vi "Sensor handling scada.vi"(7 "connect (T)":bool=TRUE, 9 "color schema":i32 step=1, 10 "AI_ALRState":i32 step=1, 11 "AI_State":i32 step=1) -> (2 "ALRSTATE":errorcluster, 3 "STATE":T1)   [LabVIEW 2019, in "Inputs.lvlib"]
uses:
  Inputs.lvlib
  Ctl/Parameter State.ctl
  Ctl/Sensor alarm scada.ctl
  Ctl/Sensor state scada.ctl
  Alarms/Alarms.lvlib
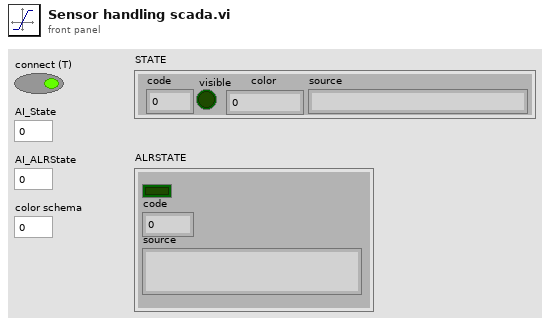
[diagram p1: front panel]
types:
  T1 = typedef "Inputs.lvlib/Parameter State.ctl" = cluster{"code":i32, "visible":bool, "color":u32, "source":string}
  T2 = typedef "Alarms.lvlib/Sensor alarm scada.ctl" = cluster{"source":string, "color":u32, "visible":bool}[]
  T3 = typedef "Inputs.lvlib/Sensor state scada.ctl" = cluster{"source":string, "color":u32, "visible":bool}[]
  T4 = cluster{"source":string, "color":u32, "visible":bool}
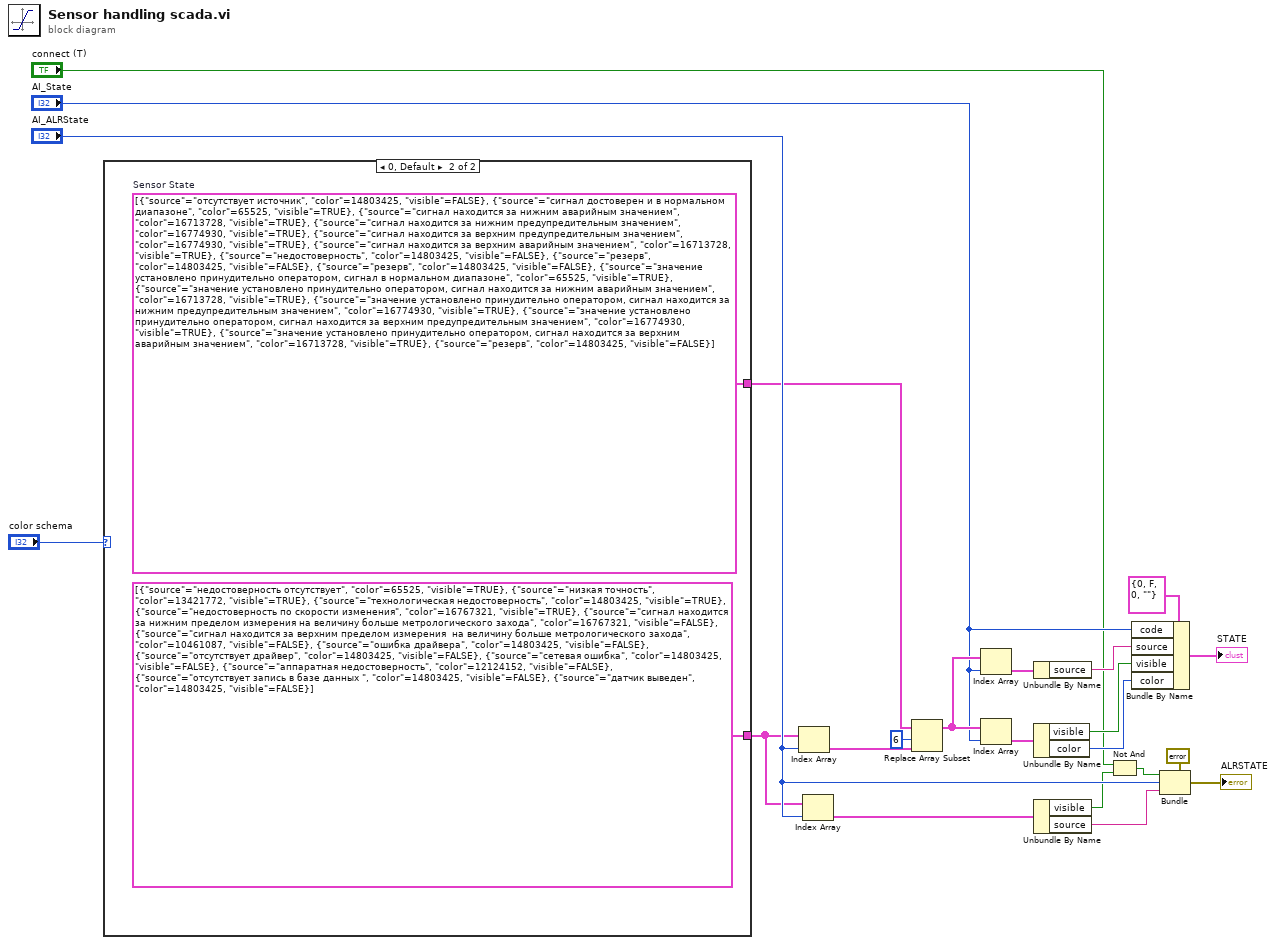
[diagram p0: block diagram]
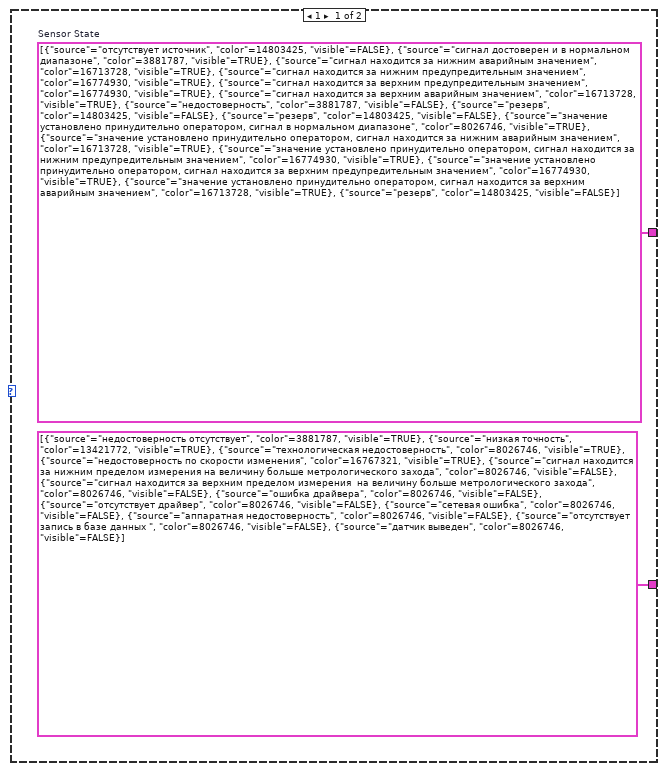
[diagram p2: hidden frame]
diagram:
  n1 = case shown="0, Default" "color schema" {
    tunnel: [w24 w26] -> w3
    tunnel: [T2 [{"source"="недостоверность отсутствует", "color"=3881787, "visible"=TRUE}, {"source"="низкая точность", "color"=13421772, "visible"=TRUE}, {"source"="технологическая недостоверность", "color"=8026746, "visible"=TRUE}, {"source"="недостоверность по скорости изменения", "color"=16767321, "visible"=TRUE}, {"source"="сигнал находится за нижним пределом измерения на величину больше метрологического захода", "color"=8026746, "visible"=FALSE}, {"source"="сигнал находится за верхним пределом измерения  на величину больше метрологического захода", "color"=8026746, "visible"=FALSE}, {"source"="ошибка драйвера", "color"=8026746, "visible"=FALSE}, {"source"="отсутствует драйвер", "color"=8026746, "visible"=FALSE}, {"source"="сетевая ошибка", "color"=8026746, "visible"=FALSE}, {"source"="аппаратная недостоверность", "color"=8026746, "visible"=FALSE}, {"source"="отсутствует запись в базе данных ", "color"=8026746, "visible"=FALSE}, {"source"="датчик выведен", "color"=8026746, "visible"=FALSE}] ("Array") T2 [{"source"="недостоверность отсутствует", "color"=65525, "visible"=TRUE}, {"source"="низкая точность", "color"=13421772, "visible"=TRUE}, {"source"="технологическая недостоверность", "color"=14803425, "visible"=TRUE}, {"source"="недостоверность по скорости изменения", "color"=16767321, "visible"=TRUE}, {"source"="сигнал находится за нижним пределом измерения на величину больше метрологического захода", "color"=16767321, "visible"=FALSE}, {"source"="сигнал находится за верхним пределом измерения  на величину больше метрологического захода", "color"=10461087, "visible"=FALSE}, {"source"="ошибка драйвера", "color"=14803425, "visible"=FALSE}, {"source"="отсутствует драйвер", "color"=14803425, "visible"=FALSE}, {"source"="сетевая ошибка", "color"=14803425, "visible"=FALSE}, {"source"="аппаратная недостоверность", "color"=12124152, "visible"=FALSE}, {"source"="отсутствует запись в базе данных ", "color"=14803425, "visible"=FALSE}, {"source"="датчик выведен", "color"=14803425, "visible"=FALSE}] ("Array")] -> w2
    frame 1 {
      w24 = T3 [{"source"="отсутствует источник", "color"=14803425, "visible"=FALSE}, {"source"="сигнал достоверен и в нормальном диапазоне", "color"=3881787, "visible"=TRUE}, {"source"="сигнал находится за нижним аварийным значением", "color"=16713728, "visible"=TRUE}, {"source"="сигнал находится за нижним предупредительным значением", "color"=16774930, "visible"=TRUE}, {"source"="сигнал находится за верхним предупредительным значением", "color"=16774930, "visible"=TRUE}, {"source"="сигнал находится за верхним аварийным значением", "color"=16713728, "visible"=TRUE}, {"source"="недостоверность", "color"=3881787, "visible"=FALSE}, {"source"="резерв", "color"=14803425, "visible"=FALSE}, {"source"="резерв", "color"=14803425, "visible"=FALSE}, {"source"="значение установлено принудительно оператором, сигнал в нормальном диапазоне", "color"=8026746, "visible"=TRUE}, {"source"="значение установлено принудительно оператором, сигнал находится за нижним аварийным значением", "color"=16713728, "visible"=TRUE}, {"source"="значение установлено принудительно оператором, сигнал находится за нижним предупредительным значением", "color"=16774930, "visible"=TRUE}, {"source"="значение установлено принудительно оператором, сигнал находится за верхним предупредительным значением", "color"=16774930, "visible"=TRUE}, {"source"="значение установлено принудительно оператором, сигнал находится за верхним аварийным значением", "color"=16713728, "visible"=TRUE}, {"source"="резерв", "color"=14803425, "visible"=FALSE}]  # Sensor State
    }
    frame 0, Default {
      w26 = T3 [{"source"="отсутствует источник", "color"=14803425, "visible"=FALSE}, {"source"="сигнал достоверен и в нормальном диапазоне", "color"=65525, "visible"=TRUE}, {"source"="сигнал находится за нижним аварийным значением", "color"=16713728, "visible"=TRUE}, {"source"="сигнал находится за нижним предупредительным значением", "color"=16774930, "visible"=TRUE}, {"source"="сигнал находится за верхним предупредительным значением", "color"=16774930, "visible"=TRUE}, {"source"="сигнал находится за верхним аварийным значением", "color"=16713728, "visible"=TRUE}, {"source"="недостоверность", "color"=14803425, "visible"=FALSE}, {"source"="резерв", "color"=14803425, "visible"=FALSE}, {"source"="резерв", "color"=14803425, "visible"=FALSE}, {"source"="значение установлено принудительно оператором, сигнал в нормальном диапазоне", "color"=65525, "visible"=TRUE}, {"source"="значение установлено принудительно оператором, сигнал находится за нижним аварийным значением", "color"=16713728, "visible"=TRUE}, {"source"="значение установлено принудительно оператором, сигнал находится за нижним предупредительным значением", "color"=16774930, "visible"=TRUE}, {"source"="значение установлено принудительно оператором, сигнал находится за верхним предупредительным значением", "color"=16774930, "visible"=TRUE}, {"source"="значение установлено принудительно оператором, сигнал находится за верхним аварийным значением", "color"=16713728, "visible"=TRUE}, {"source"="резерв", "color"=14803425, "visible"=FALSE}]  # Sensor State
    }
  }
  n2 = Index Array(array=w2, index="AI_ALRState") -> (element=w17:T4)
  n3 = Index Array(array=w2, index="AI_ALRState") -> (element=w18:T4)
  n4 = Replace Array Subset(array=w3, new element=w17, index=6) -> (w9:T3)
  n5 = Index Array(array=w9, index="AI_State") -> (element=w14:T4)
  n6 = Index Array(array=w9, index="AI_State") -> (element=w15:T4)
  n7 = Unbundle By Name(w14) -> ("source"=w16:string)
  n8 = Unbundle By Name(w15) -> ("visible"=w13:bool, "color"=w11:u32)
  n9 = Unbundle By Name(w18) -> ("visible"=w5:bool, "source"=w19:string)
  n10 = Not And(1:w5, 2:"connect (T)") -> (0:w22:bool)
  n11 = Bundle By Name(cluster=T1 {"code"=0, "visible"=FALSE, "color"=0, "source"=""} ("STATE"), "code"="AI_State", "source"=w16, "visible"=w13, "color"=w11) -> (→"STATE":T1)
  n12 = Bundle(cluster=cluster{bool, i32, "source":string} {FALSE, 0, "source"=""}, w22, "AI_ALRState", "source"=w19) -> (→"ALRSTATE":cluster{bool, i32, "source":string})
